vi "V7310.Global.vi"() -> ()   [LabVIEW 2016]
uses:
  V7310.Data.Status.ctl
  V7310.Data.Status.State.ctl
  V7310.LaserStatus.ctl
  V7310.Message.Data.ctl
  V7310.Job.Variable.ctl
  V7310.Data.Sets.ctl
  V7310.Job.Sets.ctl
panel:
  in  "IgnoreMsgID":i32[](array[numeric])
  in  "DefaultCoordinates3B":T1={"X"=-20.0, "Y"=7.7, "Angle"=-90.0}
  in  "DefaultCoordinates2B":T1={"X"=21.0, "Y"=-24.0, "Angle"=180.0}
  in  "DefaultCoordinates1B":T1={"X"=21.0, "Y"=-24.0, "Angle"=0.0}
  in  "DefaultCoordinates3A":T1={"X"=-20.0, "Y"=7.0, "Angle"=-90.0}
  in  "DefaultCoordinates2A":T1={"X"=-19.0, "Y"=-24.0, "Angle"=180.0}
  in  "DefaultCoordinates1A":T1={"X"=-19.0, "Y"=-24.0, "Angle"=0.0}
  out "Laser.Abort":bool
  in  "Laser.Sets":T2={"Address"="192.168.100.2", "Timeout_ms"=250, "ReconnectPeriod_s"=5, "JobInUse"="", "CoordinatesOffset"={"X"=0.0, "Y"=0.0}}
  out "Laser.Status":T3={"State"=enum."Init", "LaserStatus"=enum."-", "LaserStatusRaw"="", "Ref"=refnum, "RTC TS"=timestamp(0 s since 1904-01-01), "Conn TS"=timestamp(0 s since 1904-01-01), "Msg"=[], "JobInUse"="", "Jobs"=[], "Vars"=[]}
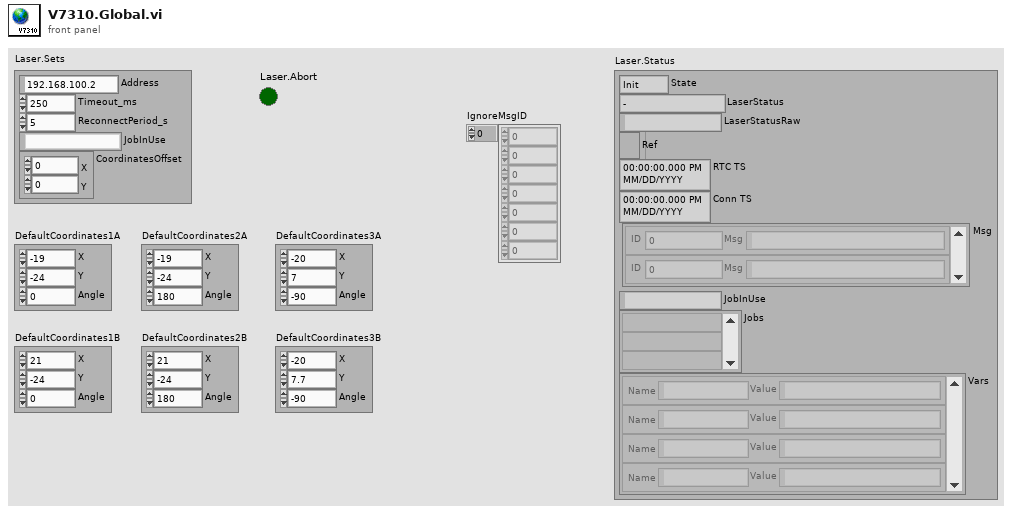
[diagram p1: front panel]
types:
  T1 = typedef "V7310.Job.Sets.ctl" = cluster{"X":dbl, "Y":dbl, "Angle":dbl}
  T2 = typedef "V7310.Data.Sets.ctl" = cluster{"Address":string, "Timeout_ms":i32, "ReconnectPeriod_s":i32, "JobInUse":string, "CoordinatesOffset":cluster{"X":dbl, "Y":dbl}}
  T3 = typedef "V7310.Data.Status.ctl" = cluster{"State":T4, "LaserStatus":T5, "LaserStatusRaw":string, "Ref":refnum<k5>, "RTC TS":timestamp, "Conn TS":timestamp, "Msg":T6[], "JobInUse":string, "Jobs":string[], "Vars":T7[]}
  T4 = typedef "V7310.Data.Status.State.ctl" = enum16{"First", "Init", "Msg", "Error", "Abort", "Idle", "Run"}
  T5 = typedef "V7310.LaserStatus.ctl" = enum16{"-", "FatalError", "Initialize", "KeySwitchOpen", "TimeoutInterlock", "InterlockOpen", "StartUp", "ShutterlockOpen", "Standby", "Ready", "PrepareForMarking", "WaitForTrigger", "Marking"}
  T6 = typedef "V7310.Message.Data.ctl" = cluster{"ID":i32, "Msg":string}
  T7 = typedef "V7310.Job.Variable.ctl" = cluster{"Name":string, "Value":string}
diagram:
